vi "Load_16bit.vi"(4 "Load in PCO Format":bool, 6 "Use Name and Number":bool, 7 "Take Full Path":bool=TRUE, 8 "error in (no error)":errorcluster, 9 "Path":path=path "\\\\Walnuss\\Silverbrick/Lab/Stefan/Data/041108/C63/s_0001.b16", 10 "Name":string, 11 "Number":i32) -> (0 "error out":errorcluster, 3 "Fluorescence Image":u16[][](graph))   [LabVIEW 2014]
panel:
  in  "File Options":T1={"Read Raw File"=0, "File Data Type"=4, "Offset to Data"=0, "Use Min Max"=enum."Don't use min max", "Optional Min Value"=0.0, "Optional Max Value"=0.0, "Byte Order"=enum."Big endian (Motorola)"} {"Optional Max Value" format="%.2f"; "Optional Min Value" format="%.2f"; "File Data Type" items=["1 bit", "2 bits", "4 bits", "8 bits", "16 bits (unsigned)", "16 bits (signed)", "16 bits (RGB chunky)", "24 bits (RGB chunky)", "24 bits (RGB planar)", "32 bits (unsigned)", "32 bits (signed)", "32 bits (RGB chunky)", "32 bits (float)", "48 bits (Complex 2x24 int)", "64 bits (Complex 2x32 float)", "32 bits (HSL)"]; "Read Raw File" items=["Don't Read Raw File ", "Read Raw File"]}
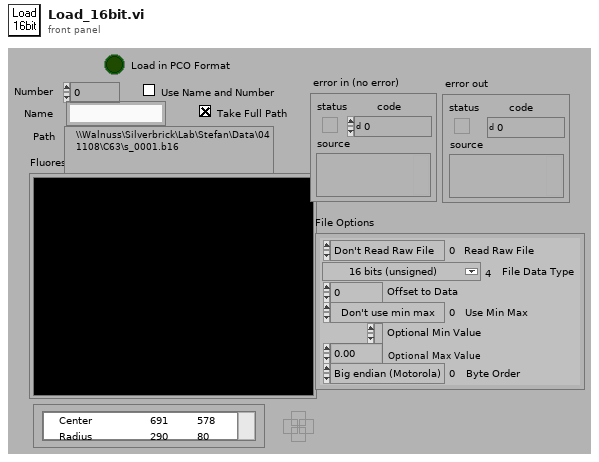
[diagram p1: front panel]
types:
  T1 = cluster{"Read Raw File":i32, "File Data Type":u32, "Offset to Data":i32, "Use Min Max":enum32{"Don't use min max", "Use file values", "Use optional values"}, "Optional Min Value":sgl, "Optional Max Value":sgl, "Byte Order":enum32{"Big endian (Motorola)", "Little endian (Intel)"}}
  T2 = typedef "IMAQ Image.ctl" = refnum<image>
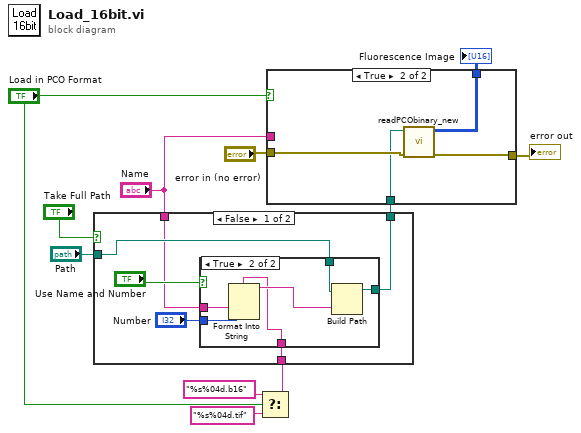
[diagram p0: block diagram]
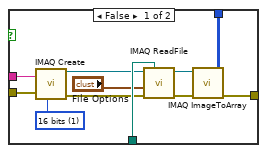
[diagram p2: hidden frame]
diagram:
  n1 = Select(t="%s%04d.b16" ("Format String"), s="Load in PCO Format", f="%s%04d.tif" ("Format String")) -> (s? t:f=w5:string)
  n2 = case shown="False" "Take Full Path" {
    tunnel: [w14 w25] -> w11
    tunnel: "Path" -> [w15 w25]
    tunnel: "Name" -> [w13 _]
    tunnel: w5 -> [w12 _]
    frame False {
      n3 = case shown="True" "Use Name and Number" {
        tunnel: "Number" -> [_ w24]
        tunnel: w15 -> [w18 w22]
        tunnel: [w18 w23] -> w14
        tunnel: w13 -> [_ w20]
        tunnel: w12 -> [_ w19]
        frame False {
        }
        frame True {
          n4 = Format Into String(format string=w19, w20, w24) -> (resulting string=w21:string)  [unwired: 2 in, 1 out]
          n5 = Build Path(base path=w22, name or relative path=w21) -> (appended path=w23:path)
        }
      }
    }
    frame True {
    }
  }
  n6 = case shown="True" "Load in PCO Format" {
    tunnel: w11 -> [w36 w38]
    tunnel: "Name" -> [w29 _]
    tunnel: [w28 w39] -> w4
    tunnel: "error in (no error)" -> [w27 w40]
    tunnel: [w26 w37] -> w1
    frame False {
      w35 = u32 1 items=["8 bits", "16 bits", "Float", "Complex", "RGB", "HSL"] ("Image Type")
      n7 = call "IMAQ Create"("Image Name"=w29, "Image Type"=w35, "error in (no error)"=w27) -> ("New Image"=w33:T2, "error out"=w34:errorcluster)  [unwired: 2 in]
      n8 = call "IMAQ ReadFile"("File Path"=w36, "error in (no error)"=w34, "File Options"="File Options", "Image"=w33) -> ("error out"=w31:errorcluster, "Image Out"=w30:T2)  [unwired: 3 in, 3 out]
      n9 = call "IMAQ ImageToArray"("error in (no error)"=w31, "Image"=w30) -> ("error out"=w28:errorcluster, "Image Pixels (I16)"=w26:i16[][])  [unwired: 2 in, 3 out]
    }
    frame True {
      n10 = call "readPCObinary_new.vi"("error in (no error)"=w40, "Image Path"=w38) -> ("error out"=w39:errorcluster, "Image"=w37:u16[][])  [unwired: 8 in]
    }
  }
  "error out" <- w4
  "Fluorescence Image" <- w1
